vi "Save DAC Configuration.vi"(8 "error in":errorcluster, 10 "Config File refnum in":T1, 11 "DAC Shunt dU in":refnum<class "DAC Shunt dU.lvclass">) -> (0 "error out":errorcluster, 2 "Config File refnum out":T1, 3 "DAC Shunt dU out":refnum<class "DAC Shunt dU.lvclass">)   [LabVIEW 2019, in "DAC.lvlib" / "DAC Shunt dU.lvclass"]
uses:
  DAC Shunt dU.lvclass
  C:/Users/krio/Documents/LV_Projects/TestStand/App/DAC/DAC.lvclass
  <vilib>/Utility/config.llb/Config Data RefNum.ctl
  DAC.lvclass/DAC.ctl
  DAC Shunt dU.lvclass/DAC Shunt dU.ctl
  <vilib>/Utility/config.llb/Write Key (String).vi
  <vilib>/Utility/config.llb/Write Key (Double).vi
  DAC.lvclass
  <vilib>/Utility/config.llb/NI_LVConfig.lvlib
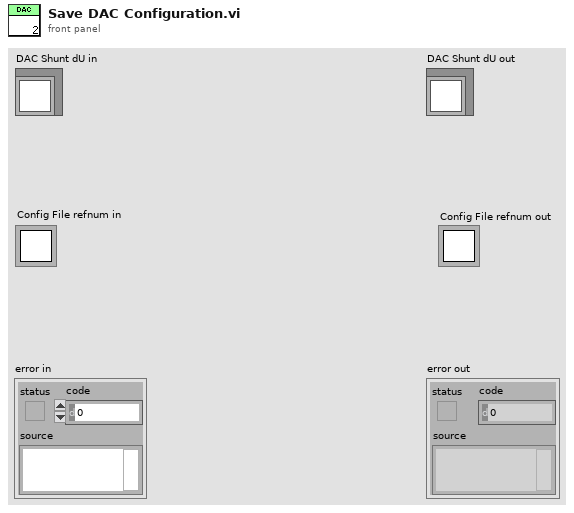
[diagram p1: front panel]
types:
  T1 = typedef "NI_LVConfig.lvlib/Config Data RefNum.ctl" = refnum<k1>
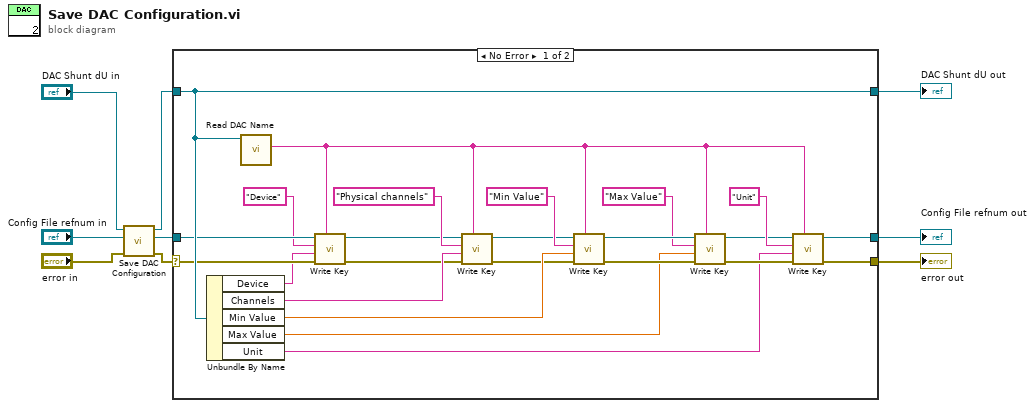
[diagram p0: block diagram]
diagram:
  n1 = call-parent "Save DAC Configuration.vi"("error in"="error in", "Config File refnum in"="Config File refnum in", "DAC in"="DAC Shunt dU in") -> ("error out"=w4:errorcluster, "Config File refnum out"=w5:T1, "DAC out"=w6:refnum<class "DAC Shunt dU.lvclass">)  [unwired: 6 in]
  n2 = case shown="No Error" w4 {
    selector: w4 -> [w21 w36]
    tunnel: [w12 w36] -> w1
    tunnel: [w27 w35] -> w3
    tunnel: w6 -> [w27 w35]
    tunnel: w5 -> [w22 w34]
    tunnel: [w14 w34] -> w2
    frame No Error {
      n3 = Unbundle By Name(w27) -> ("Device"=w17:string, "Channels"=w23:string, "Min Value"=w29:dbl, "Max Value"=w28:dbl, "Unit"=w11:string)
      n4 = call "Read DAC Name.vi"("DAC in"=w27) -> ("DAC Name"=w10:string)  [unwired: 8 in, 2 out]
      n5 = call-poly <vilib>:"Write Key.vi"("section"=w10, "error in (no error)"=w21, "value"=w17, "key"="Device", "refnum"=w22) -> ("error out"=w19:errorcluster, "refnum out"=w20:T1)  [unwired: 4 in, 1 out]
      n6 = call-poly <vilib>:"Write Key.vi"("section"=w10, "error in (no error)"=w19, "value"=w23, "key"="Physical channels", "refnum"=w20) -> ("error out"=w25:errorcluster, "refnum out"=w26:T1)  [unwired: 4 in, 1 out]
      n7 = call-poly <vilib>:"Write Key.vi"("section"=w10, "error in (no error)"=w25, "value"=w29, "key"="Min Value", "refnum"=w26) -> ("error out"=w32:errorcluster, "refnum out"=w33:T1)  [unwired: 4 in, 1 out]
      n8 = call-poly <vilib>:"Write Key.vi"("section"=w10, "error in (no error)"=w32, "value"=w28, "key"="Max Value", "refnum"=w33) -> ("error out"=w13:errorcluster, "refnum out"=w15:T1)  [unwired: 4 in, 1 out]
      n9 = call-poly <vilib>:"Write Key.vi"("section"=w10, "error in (no error)"=w13, "value"=w11, "key"="Unit", "refnum"=w15) -> ("error out"=w12:errorcluster, "refnum out"=w14:T1)  [unwired: 4 in, 1 out]
    }
    frame Error {
    }
  }
  "error out" <- w1
  "DAC Shunt dU out" <- w3
  "Config File refnum out" <- w2
